vi "Update Tags.vi"(8 "error in (no error)":errorcluster, 9 "Child Text":string[][](array[string]), 10 "Tag":string[](array[string]), 11 "Tag Tree Helper In":refnum<class "Tag Tree Helper.lvclass">) -> (0 "error out":errorcluster, 3 "Tag Tree Helper Out":refnum<class "Tag Tree Helper.lvclass">)   [LabVIEW 2020, in "Tag Tree Helper.lvclass"]
uses:
  Tag Tree Helper.lvclass
  Tag Tree Helper.lvclass/Tag Tree Helper.ctl
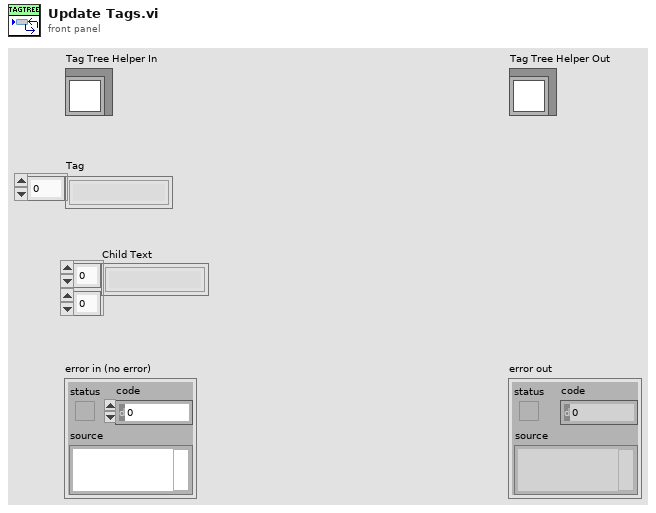
[diagram p1: front panel]
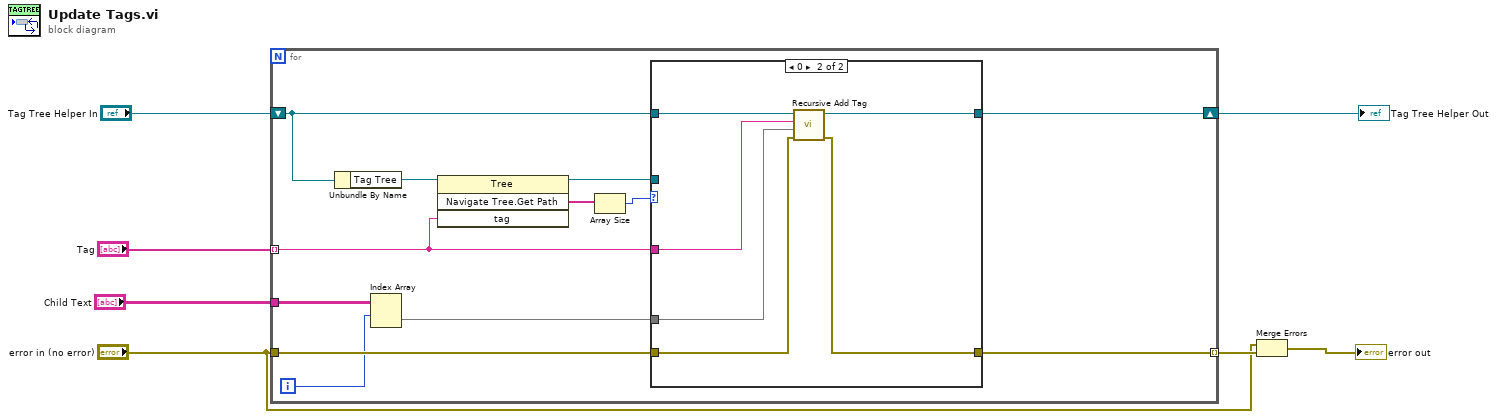
[diagram p0: block diagram]
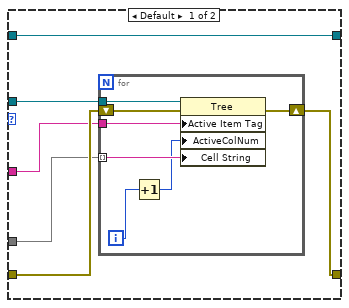
[diagram p2: hidden frame]
diagram:
  n1 = for {
    tunnel: "Tag" -> [w10] mode=indexing
    shift-right: [w11] -> w5
    shift-left: "Tag Tree Helper In" -> [w12]
    tunnel: "error in (no error)" -> [w17]
    tunnel: [w18] -> w4 mode=indexing
    tunnel: "Child Text" -> [w16]
    i -> [w15]
    n2 = Unbundle By Name(w12) -> ("Tag Tree"=w19:refnum<vi>)
    n3 = Index Array(array=w16, index (row)=w15) -> (element=w14:string[])  [unwired: 1 in]
    n4 = invoke on="Invoke Node" class="Tree" method="Navigate Tree.Get Path"(reference=w19, "tag"=w10) -> (reference out=w13:refnum<vi>, "Navigate Tree:Get Path"=w8:string[])  [unwired: 2 in, 2 out]
    n5 = Array Size(array=w8) -> (size(s)=w9:i32)
    n6 = case shown="0" w9 {
      tunnel: [w25 w33] -> w18
      tunnel: w17 -> [w24 w34]
      tunnel: w14 -> [w23 w35]
      tunnel: w13 -> [w22 _]
      tunnel: w10 -> [w21 w36]
      tunnel: w12 -> [w20 w38]
      tunnel: [w20 w37] -> w11
      frame Default {
        n7 = for {
          tunnel: w22 -> [w32]
          tunnel: w21 -> [w29]
          shift-right: [w31] -> w25
          shift-left: w24 -> [w30]
          tunnel: w23 -> [w28] mode=indexing
          i -> [w27]
          n8 = Increment(x=w27) -> (x+1=w26:i32)
          n9 = property on="Property Node" class="Tree"(reference=w32, error in=w30, "Active Item Tag"=w29, "ActiveColNum"=w26, "Cell String"=w28) -> (error out=w31:errorcluster)  [unwired: 1 out]
        }
      }
      frame 0 {
        n10 = call "Recursive Add Tag.vi"("error in (no error)"=w34, "Child Text"=w35, "Tag"=w36, "Tag Tree Helper In"=w38) -> ("error out"=w33:errorcluster, "Tag Tree Helper Out"=w37:refnum<class "Tag Tree Helper.lvclass">)  [unwired: 6 in]
      }
    }
  }
  "Tag Tree Helper Out" <- w5
  n11 = Merge Errors("error in (no error)", w4) -> (→"error out":errorcluster)
